vi "save config.vi"(8 "error in (no error)":errorcluster, 10 "TABLE":string="power_environment_monitoring", 11 "VI引用句柄":refnum<vi>) -> (0 "error out":errorcluster)   [LabVIEW 2016]
uses:
  <userlib>/_LVST/sqlite_api/Core/Tables/SQLite_Create Table.vi
  <userlib>/_LVST/sqlite_api/Core/Insert/SQLite_Upsert.vi
  <vilib>/Utility/sysdir.llb/System Directory Type.ctl
panel:
  out "数组":string[][](array[string])
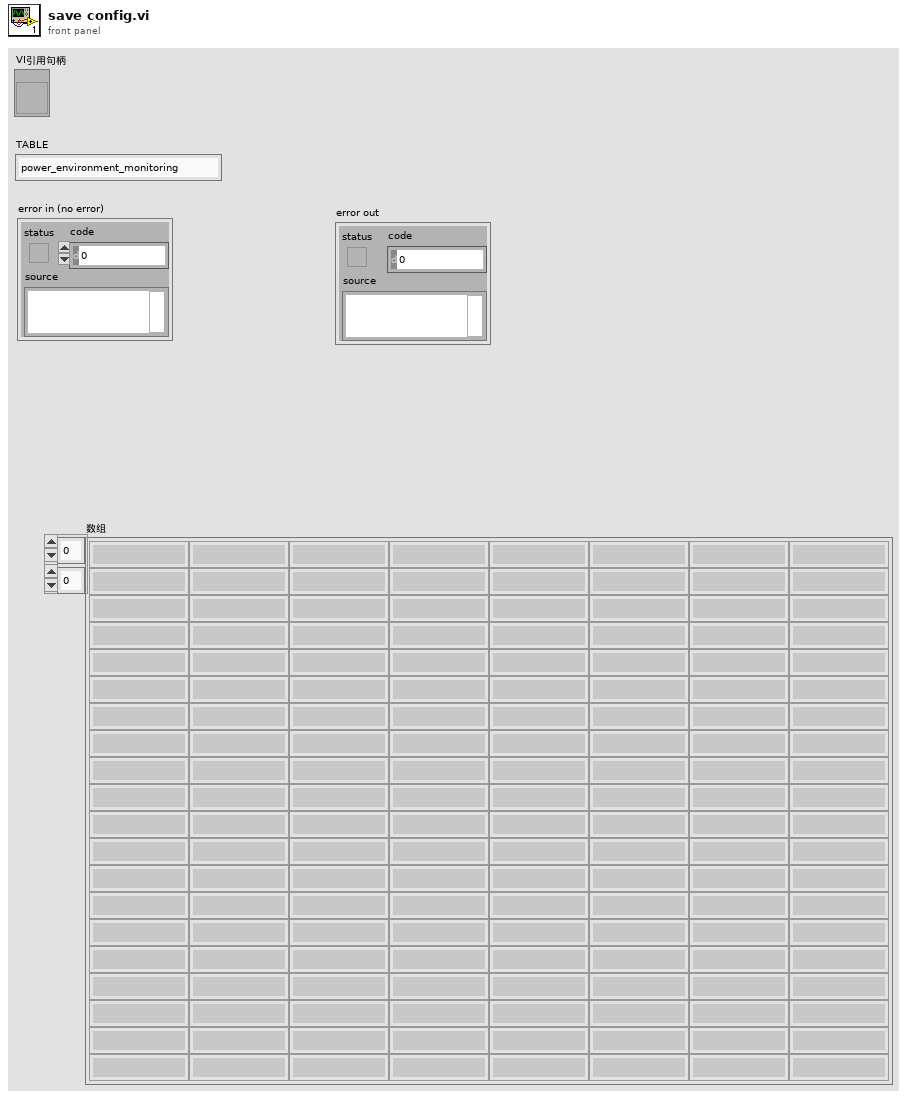
[diagram p1: front panel]
types:
  T1 = typedef "System Directory Type.ctl" = i32
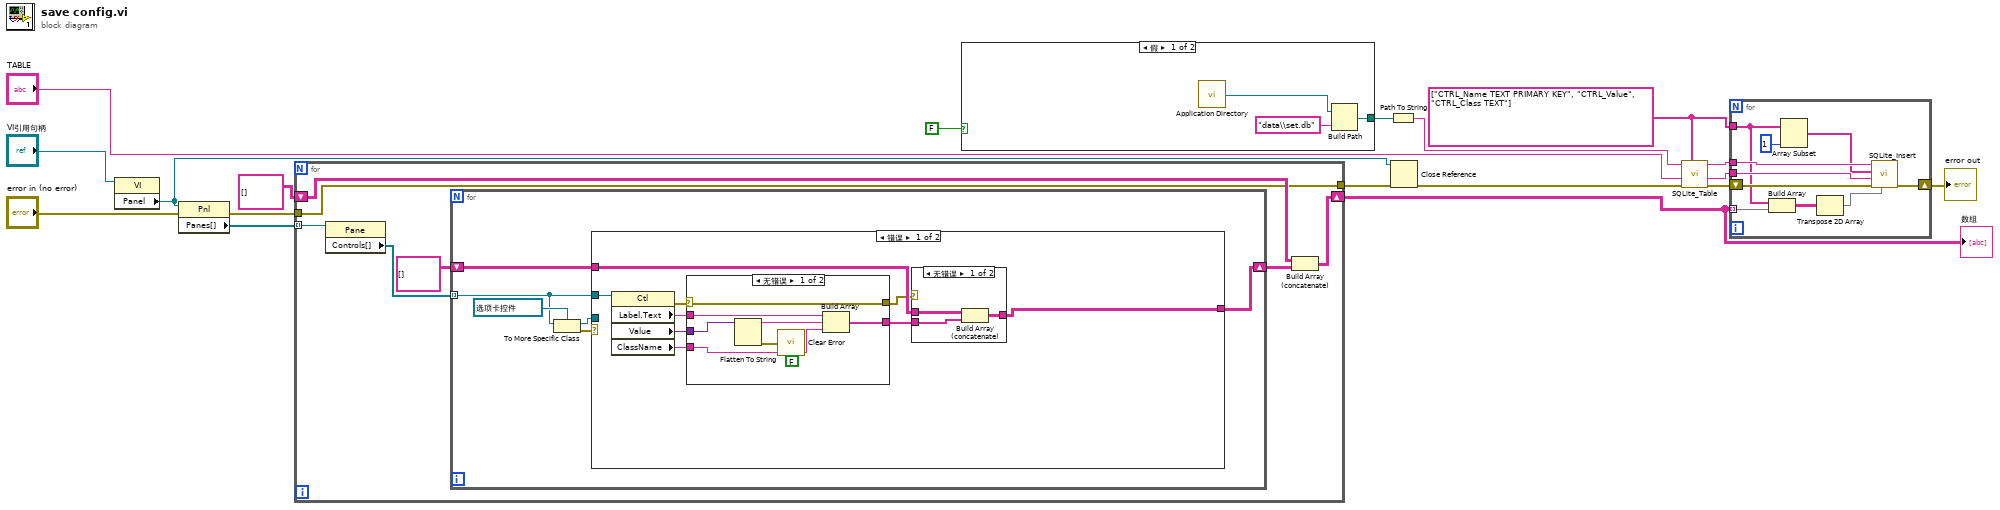
[diagram p0: block diagram]
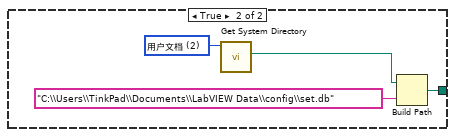
[diagram p2: hidden frame]
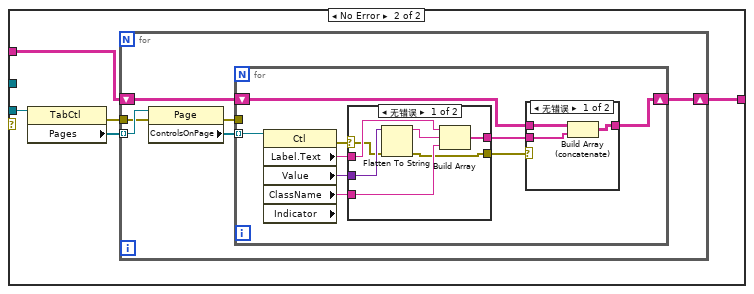
[diagram p5: hidden frame]
diagram:
  w12 = string[] ["CTRL_Name TEXT PRIMARY KEY", "CTRL_Value", "CTRL_Class TEXT"] ("Column")
  n1 = property class="VI"(reference="VI引用句柄") -> ("Panel"=w7:refnum<vi>)  [unwired: 1 in, 2 out]
  n2 = property class="Pnl"(reference=w7, error in="error in (no error)") -> (error out=w6:errorcluster, "Panes[]"=w11:refnum<vi>[])  [unwired: 1 out]
  n3 = for {
    tunnel: w11 -> [w24] mode=indexing
    shift-right: [w23] -> w8
    shift-left: string[][] [] -> [w21]
    tunnel: w6 -> [w19]
    tunnel: [w19] -> w5
    n4 = property class="Pane"(reference=w24) -> ("Controls[]"=w25:refnum<vi>[])  [unwired: 1 in, 2 out]
    n5 = for {
      tunnel: w25 -> [w27] mode=indexing
      shift-right: [w30] -> w22
      shift-left: string[][] [] -> [w29]
      n6 = To More Specific Class(target class=refnum<vi> refnum ("Tabs"), reference=w27) -> (specific class reference=w31:refnum<vi>, error out=w26:errorcluster)  [unwired: 1 in]
      n7 = case shown="错误" w26 {
        tunnel: w31 -> [_ w57]
        tunnel: [w40 w54] -> w30
        tunnel: w29 -> [w39 w53]
        tunnel: w27 -> [w35 _]
        frame Error {
          n8 = property class="Ctl"(reference=w35) -> (error out=w33:errorcluster, "Label.Text"=w34:string, "Value"=w37:variant, "ClassName"=w38:string)  [unwired: 1 in, 1 out]
          n9 = case shown="无错误" w33 {
            selector: w33 -> [w49 w52]
            tunnel: w34 -> [w45 _]
            tunnel: w37 -> [w48 _]
            tunnel: [w51 _] -> w32
            tunnel: w38 -> [w50 _]
            tunnel: [w49 w52] -> w36
            frame No Error {
              (unwired) FALSE ("预置数组或字符串大小？ (T)")
              n10 = Flatten To String(anything=w48) -> (data string=w47:string, error out=w46:errorcluster)  [unwired: 3 in, 1 out]
              n11 = call <userlib>:"Clear Error.vi"("error in (no error)"=w46) -> ()  [unwired: 4 in, 1 out]
              n12 = Build Array(w45, w47, w50) -> (w51:string[])
            }
            frame Error {
            }
          }
          n13 = case shown="无错误" w36 {
            tunnel: w32 -> [w43 _]
            tunnel: [w42 w44] -> w40
            tunnel: w39 -> [w41 w44]
            frame No Error {
              n14 = Build Array (concatenate)(w41, w43) -> (w42:string[][])
            }
            frame Error {
            }
          }
        }
        frame No Error {
          n15 = property class="TabCtl"(reference=w57) -> (error out=w55:errorcluster, "Pages"=w56:refnum<vi>[])  [unwired: 1 in, 1 out]
          n16 = for {
            tunnel: w56 -> [w63] mode=indexing
            tunnel: w55 -> [w61]
            shift-right: [w59] -> w54
            shift-left: w53 -> [w58]
            n17 = property class="Page"(reference=w63, error in=w61) -> (error out=w62:errorcluster, "ControlsOnPage"=w60:refnum<vi>[])  [unwired: 1 out]
            n18 = for {
              tunnel: w62 -> [_]
              tunnel: w60 -> [w66] mode=indexing
              shift-right: [w72] -> w59
              shift-left: w58 -> [w71]
              n19 = property class="Ctl" props=["Label", "Text", "Value", "ClassName", "Indicator"](reference=w66) -> (error out=w67:errorcluster, "Label.Text"=w68:string, "Value"=w69:variant, "ClassName"=w70:string)  [unwired: 1 in, 2 out]
              n20 = case shown="无错误" w67 {
                selector: w67 -> [w74 w80]
                tunnel: w68 -> [w79 _]
                tunnel: w69 -> [w76 _]
                tunnel: [w78 _] -> w65
                tunnel: w70 -> [w77 _]
                tunnel: [w73 w80] -> w64
                frame No Error {
                  n21 = Flatten To String(anything=w76, error in (no error)=w74) -> (data string=w75:string, error out=w73:errorcluster)  [unwired: 2 in, 1 out]
                  n22 = Build Array(w79, w75, w77) -> (w78:string[])
                }
                frame Error {
                }
              }
              n23 = case shown="无错误" w64 {
                tunnel: w65 -> [w83 _]
                tunnel: [w82 w84] -> w72
                tunnel: w71 -> [w81 w84]
                frame No Error {
                  n24 = Build Array (concatenate)(w81, w83) -> (w82:string[][])
                }
                frame Error {
                }
              }
            }
          }
        }
      }
    }
    n25 = Build Array (concatenate)(w21, w22) -> (w23:string[][])
  }
  "数组" <- w8
  n26 = case shown="假" FALSE {
    tunnel: [w85 w88] -> w2
    frame False {
      n27 = call <vilib>:"Application Directory.vi"() -> ("Application Directory"=w87:path)
      n28 = Build Path(base path=w87, name or relative path="data\\set.db" ("名称或相对路径")) -> (appended path=w85:path)
    }
    frame True {
      w91 = T1 2 items=["用户目录"=0, "用户桌面"=1, "用户文档"=2, "用户应用程序数据"=3, "用户设置"=4, "用户临时目录"=5, "公共文档"=6, "公共应用程序数据"=7, "公共设置"=8, "公共缓存"=13, "系统核心库"=9, "系统安装库"=10, "应用程序文件"=11, "启动盘根目录"=12] ("system directory type")
      n29 = call <vilib>:"Get System Directory.vi"("system directory type"=w91) -> ("system directory"=w89:path)  [unwired: 10 in]
      n30 = Build Path(base path=w89, name or relative path="C:\\Users\\TinkPad\\Documents\\LabVIEW Data\\config\\set.db" ("名称或相对路径")) -> (appended path=w88:path)
    }
  }
  n31 = Path To String(path=w2) -> (string=w15:string)
  n32 = Close Reference(reference=w7, error in (no error)=w5) -> (error out=w14:errorcluster)
  n33 = call-poly <userlib>:"SQLite_Table.vi"("DB Path"=w15, "Table Name"="TABLE", "error in (no error)"=w14, "Columns"=w12) -> ("DB Path Out"=w17:string, "Table Name Out"=w16:string, "error out"=w18:errorcluster)  [unwired: 4 in]
  n34 = for {
    tunnel: w17 -> [w99]
    tunnel: w16 -> [w98]
    tunnel: w8 -> [w97] mode=indexing
    tunnel: w12 -> [w94]
    shift-right: [w101] -> w13
    shift-left: w18 -> [w100]
    n35 = Build Array(w94, w97) -> (w96:string[][])
    n36 = Array Subset(array=w94, length=1) -> (w93:string[])  [unwired: 1 in]
    n37 = Transpose 2D Array(2D array=w96) -> (transposed array=w95:string[][])
    n38 = call-poly <userlib>:"SQLite_Insert.vi"("Column/Value Pairs"=w95, "error in"=w100, "Table Name"=w98, "Constraint Columns"=w93, "DB Path"=w99) -> ("error out"=w101:errorcluster)  [unwired: 2 in, 2 out]
  }
  "error out" <- w13
